vi "Get Wheel Parameter by Name.vi"(8 "error in (no error)":errorcluster, 10 "parameter name":string, 11 "wheel in":refnum<class "NI_Robotics_Caster Wheel.lvclass">) -> (0 "error out":errorcluster, 1 "found?":bool, 2 "parameter value":variant, 3 "wheel out":refnum<class "NI_Robotics_Caster Wheel.lvclass">)   [LabVIEW 2017, in "NI_Robotics_Caster Wheel.lvclass"]
uses:
  <vilib>/robotics/Steering/Caster Wheel/NI_Robotics_Caster Wheel.lvclass
  <vilib>/robotics/Steering/Caster Wheel/NI_Robotics_Caster Wheel.lvclass/NI_Robotics_Caster Wheel.ctl
  <vilib>/robotics/Steering/Wheel/NI_Robotics_Wheel.lvclass
  <vilib>/robotics/Actuation/Motor Communication/NI_Robotics_Motor Communication.lvclass
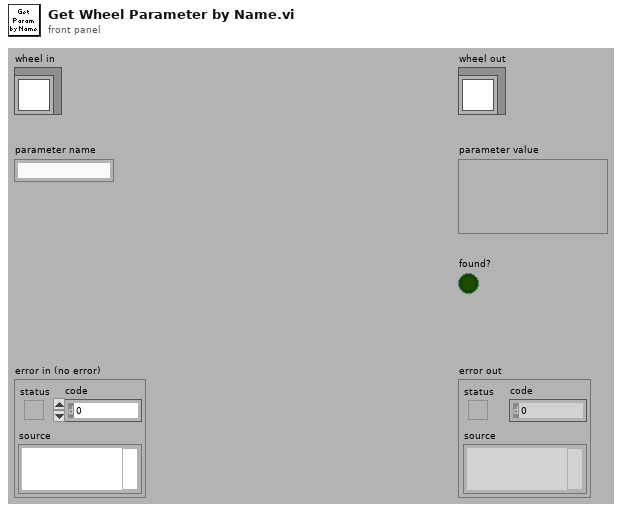
[diagram p1: front panel]
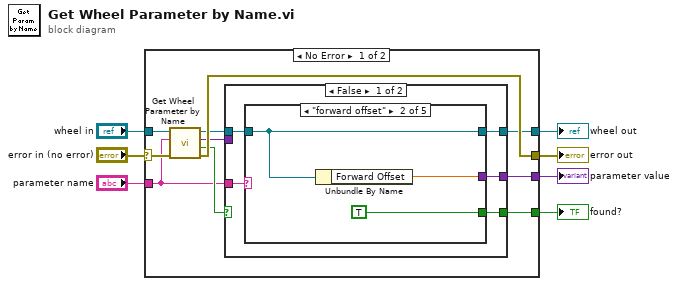
[diagram p0: block diagram]
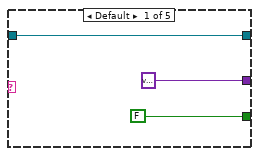
[diagram p2: hidden frame]
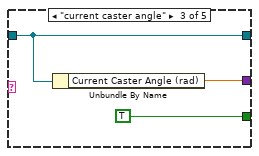
[diagram p3: hidden frame]
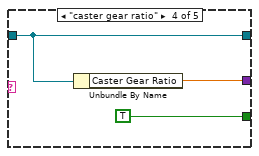
[diagram p4: hidden frame]
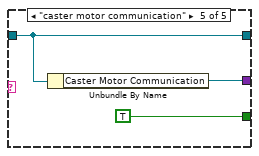
[diagram p5: hidden frame]
diagram:
  n1 = case shown="No Error" "error in (no error)" {
    selector: "error in (no error)" -> [w15 w41]
    tunnel: [w17 w41] -> w7
    tunnel: [w9 _] -> w6
    tunnel: [w10 _] -> w5
    tunnel: [w11 w42] -> w4
    tunnel: "parameter name" -> [w8 _]
    tunnel: "wheel in" -> [w16 w42]
    frame No Error {
      n2 = call-parent "Get Wheel Parameter by Name.vi"("error in (no error)"=w15, "parameter name"=w8, "wheel in"=w16) -> ("error out"=w17:errorcluster, "found?"=w14:bool, "parameter value"=w13:variant, "wheel out"=w12:refnum<class "NI_Robotics_Caster Wheel.lvclass">)  [unwired: 5 in]
      n3 = case shown="False" w14 {
        selector: w14 -> [_ w38]
        tunnel: w13 -> [_ w39]
        tunnel: w12 -> [w21 w40]
        tunnel: [w20 w40] -> w11
        tunnel: [w19 w39] -> w10
        tunnel: [w18 w38] -> w9
        tunnel: w8 -> [w22 _]
        frame False {
          n4 = case shown="\"forward offset\"" w22 {
            tunnel: w21 -> [w25 w28 w31 w34 w37]
            tunnel: [w25 w28 w31 w34 w37] -> w20
            tunnel: [variant ("parameter value") w27 w30 w33 w36] -> w19
            tunnel: [FALSE TRUE TRUE TRUE TRUE] -> w18
            frame Default {
            }
            frame "forward offset" {
              n5 = Unbundle By Name(w28) -> ("Forward Offset"=w27:dbl)
            }
            frame "current caster angle" {
              n6 = Unbundle By Name(w31) -> ("Current Caster Angle (rad)"=w30:dbl)
            }
            frame "caster gear ratio" {
              n7 = Unbundle By Name(w34) -> ("Caster Gear Ratio"=w33:dbl)
            }
            frame "caster motor communication" {
              n8 = Unbundle By Name(w37) -> ("Caster Motor Communication"=w36:refnum<class "NI_Robotics_Motor Communication.lvclass">)
            }
          }
        }
        frame True {
        }
      }
    }
    frame Error {
    }
  }
  "error out" <- w7
  "wheel out" <- w4
  "parameter value" <- w5
  "found?" <- w6
